vi "Discovery Cluster Id.vi"() -> (3 "nidiscovery_clusterid":string="NIDISCOVERY_CLUSTERID")   [LabVIEW 2024]
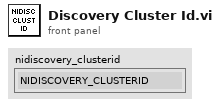
[diagram p1: front panel]
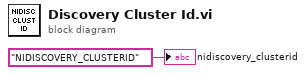
[diagram p0: block diagram]
diagram:
  "nidiscovery_clusterid" <- "NIDISCOVERY_CLUSTERID"
